vi "CVT Double IndexRead.vi"(3 "error in (no error)":errorcluster, 5 "Tag Index":i32) -> (0 "error out":errorcluster, 1 "Value":dbl)   [LabVIEW 2010]
uses:
  _SubVIs/TypeDefs/cvt_MemBlock Methods.ctl
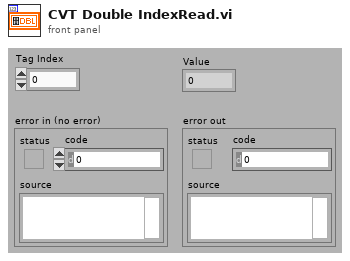
[diagram p1: front panel]
types:
  T1 = typedef "cvt_MemBlock Methods.ctl" = enum16{"init", "read", "readall", "write"}
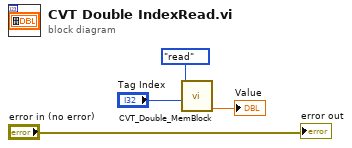
[diagram p0: block diagram]
diagram:
  n1 = call "CVT_Double_MemBlock.vi"("Index"="Tag Index", "Method"=cvt_MemBlock_Methods."read" ("function")) -> ("Value"=→"Value":dbl)  [unwired: 2 in, 7 out]
  "error out" <- "error in (no error)"
